vi "tool_Unicode_Display String Text.vi"(5 "Interpret as Unicode (T)":bool, 6 "error in":errorcluster, 8 "String Value":string, 9 "String Control Reference":refnum<vi>) -> (0 "error out":errorcluster, 3 "String Control Reference":refnum<vi>)   [LabVIEW 2020]
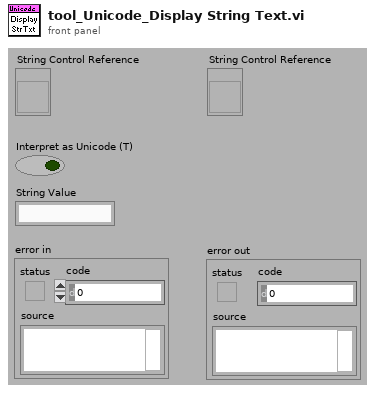
[diagram p1: front panel]
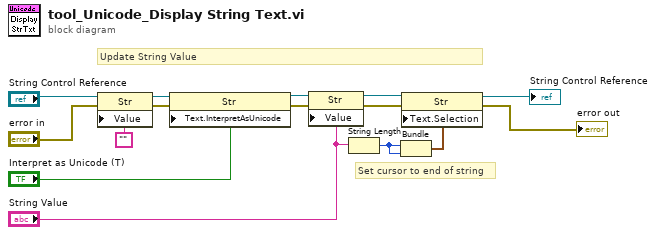
[diagram p0: block diagram]
diagram:
  # "Update String Value"
  # "Set cursor to end of string"
  n1 = property class="Str"(reference="String Control Reference", error in="error in", "Value"="") -> (reference out=w3:refnum<vi>, error out=w10:errorcluster)
  n2 = property class="Str"(reference=w3, error in=w10, "Text.InterpretAsUnicode"="Interpret as Unicode (T)") -> (reference out=w12:refnum<vi>, error out=w11:errorcluster)
  n3 = property class="Str"(reference=w12, error in=w11, "Value"="String Value") -> (reference out=w4:refnum<vi>, error out=w5:errorcluster)
  n4 = String Length(string="String Value") -> (length=w8:i32)
  n5 = Bundle(w8, w8) -> (w9:cluster{i32, i32})  [unwired: 1 in]
  n6 = property class="Str"(reference=w4, error in=w5, "Text.Selection"=w9) -> (reference out=→"String Control Reference":refnum<vi>, error out=→"error out":errorcluster)
